vi "Result.vi"(2 "Blackjack odds":dbl, 3 "Bet":dbl, 4 "Chips before":dbl, 5 "Result":i16) -> (0 "String":string, 1 "Chips now":dbl)   [LabVIEW 2018]
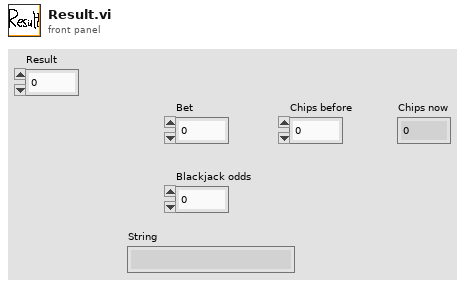
[diagram p1: front panel]
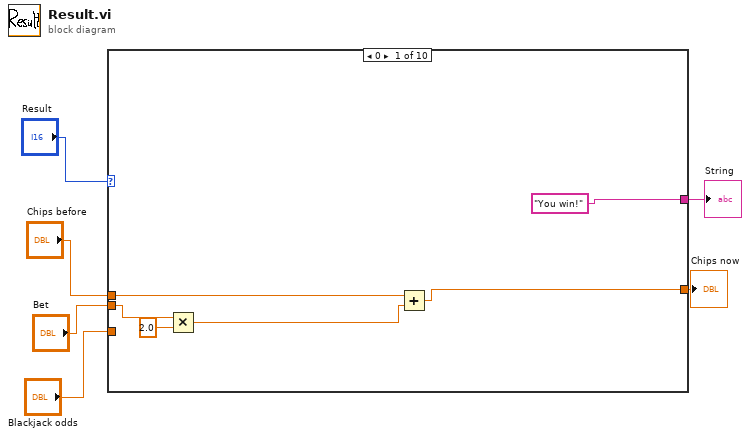
[diagram p0: block diagram]
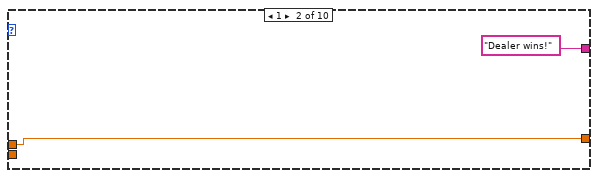
[diagram p2: hidden frame]
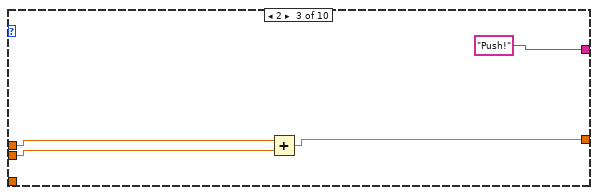
[diagram p3: hidden frame]
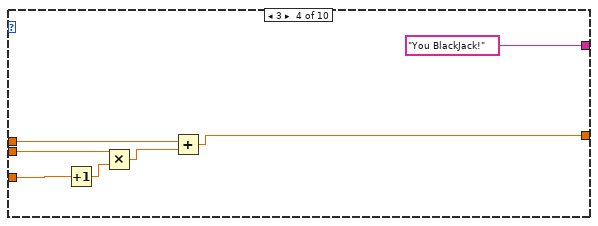
[diagram p4: hidden frame]
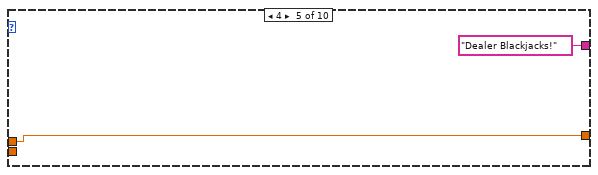
[diagram p5: hidden frame]
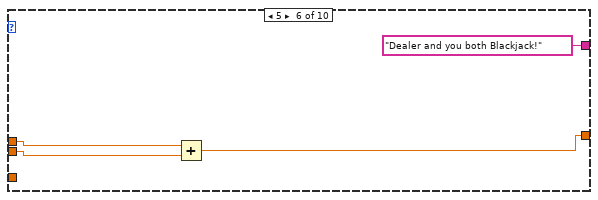
[diagram p6: hidden frame]
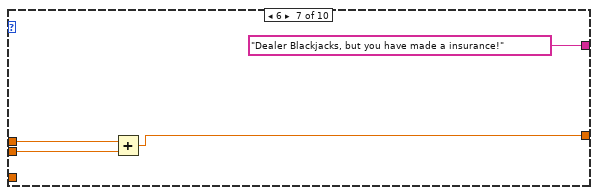
[diagram p7: hidden frame]
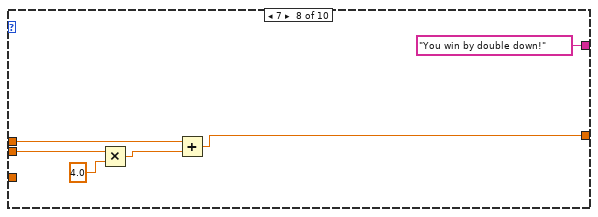
[diagram p8: hidden frame]
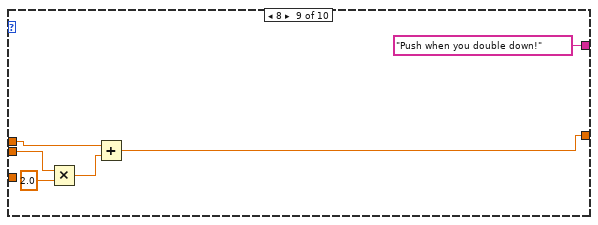
[diagram p9: hidden frame]
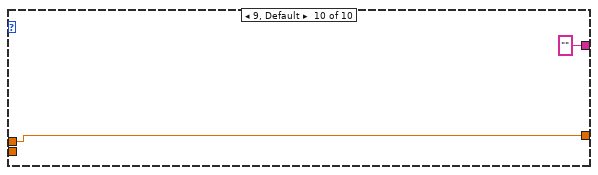
[diagram p10: hidden frame]
diagram:
  n1 = case shown="0" "Result" {
    tunnel: ["You win!" "Dealer wins!" "Push!" "You BlackJack!" "Dealer Blackjacks!" "Dealer and you both Blackjack!" "Dealer Blackjacks, but you have made a insurance!" "You win by double down!" "Push when you double down!" ""] -> w5
    tunnel: "Chips before" -> [w11 w13 w17 w22 w26 w30 w34 w37 w44 w49]
    tunnel: "Bet" -> [w9 _ w16 w24 _ w29 w33 w40 w46 _]
    tunnel: [w10 w13 w15 w21 w26 w28 w32 w36 w43 w49] -> w2
    tunnel: "Blackjack odds" -> [_ _ _ w20 _ _ _ _ _ _]
    frame 0 {
      n2 = Multiply(x=w9, y=2.0) -> (x*y=w7:dbl)
      n3 = Add(x=w11, y=w7) -> (x+y=w10:dbl)
    }
    frame 1 {
    }
    frame 2 {
      n4 = Add(x=w17, y=w16) -> (x+y=w15:dbl)
    }
    frame 3 {
      n5 = Increment(x=w20) -> (x+1=w19:dbl)
      n6 = Multiply(x=w24, y=w19) -> (x*y=w23:dbl)
      n7 = Add(x=w22, y=w23) -> (x+y=w21:dbl)
    }
    frame 4 {
    }
    frame 5 {
      n8 = Add(x=w30, y=w29) -> (x+y=w28:dbl)
    }
    frame 6 {
      n9 = Add(x=w34, y=w33) -> (x+y=w32:dbl)
    }
    frame 7 {
      n10 = Multiply(x=w40, y=4.0) -> (x*y=w38:dbl)
      n11 = Add(x=w37, y=w38) -> (x+y=w36:dbl)
    }
    frame 8 {
      n12 = Multiply(x=w46, y=2.0) -> (x*y=w45:dbl)
      n13 = Add(x=w44, y=w45) -> (x+y=w43:dbl)
    }
    frame 9, Default {
    }
  }
  "String" <- w5
  "Chips now" <- w2
